vi "SQL_writeV2.vi"() -> ()   [LabVIEW 2019]
uses:
  <vilib>/OPCUA/NI OPC UA Client.lvlib
panel:
  out "date/time string":string
  in  "stop":bool
  in  "server endpoint URL":string
  # "OPC-UA Settings"
  # "SQL-Write Settings"
  # "Inputs:"
  # "Outputs"
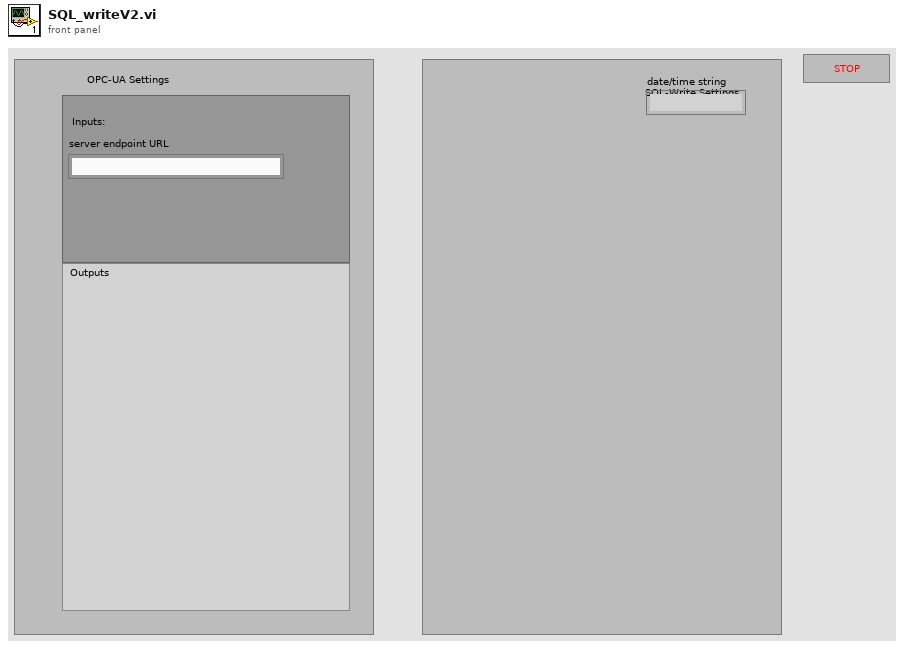
[diagram p1: front panel]
types:
  T1 = cluster{"message mode":enum16{"None", "Sign", "Sign and Encrypt"}, "security":enum16{"Basic256", "Basic128Rsa15"}}
  T2 = typedef "OPC UA Client Refnum.ctl" = refnum<k21>
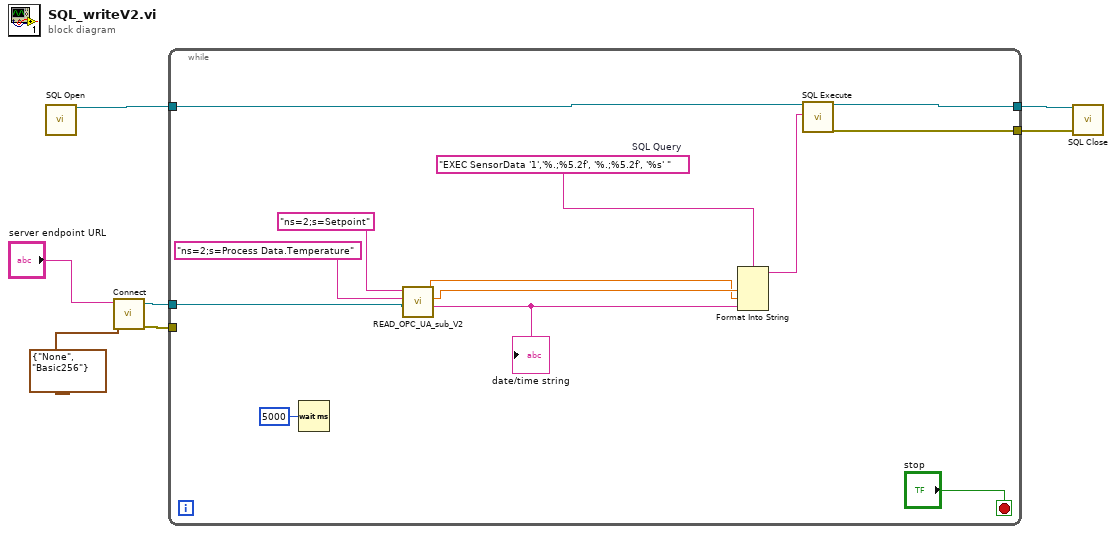
[diagram p0: block diagram]
diagram:
  n1 = call <vilib>:"SQL Open.vi"() -> ("ConnectionString In"=w2:string, "Connection Out"=w8:refnum<k7>)  [unwired: 17 in, 1 out]
  n2 = call <vilib>:"Connect.vi"("security policy"=T1 {"message mode"=enum."None", "security"=enum."Basic256"}, "server endpoint URL"="server endpoint URL") -> ("error out"=w3:errorcluster, "OPC UA client refnum out"=w4:T2)  [unwired: 7 in, 1 out]
  n3 = while {
    tunnel: w8 -> [w14]
    tunnel: [w13] -> w7
    tunnel: w4 -> [w17]
    tunnel: w3 -> [_]
    tunnel: [w12] -> w1
    stop <- "stop" stop-if-true
    w15 = "EXEC SensorData '1','%.;%5.2f', '%.;%5.2f', '%s' "  # SQL Query
    n4 = Wait (ms)(milliseconds to wait=u32 5000) -> ()  [unwired: 1 out]
    n5 = call "READ_OPC_UA_sub_V2.vi"("Node Id(setpoint)"="ns=2;s=Setpoint", "Node Id(temperature)"="ns=2;s=Process Data.Temperature", "OPC UA client refnum in"=w17) -> ("Temperature Value[C]"=w10:dbl, "Setpoint[C]"=w11:dbl, "date/time string"=w9:string)  [unwired: 5 in]
    "date/time string" <- w9
    n6 = Format Into String(format string=w15, w11, w10, w9) -> (resulting string=w16:string)  [unwired: 2 in, 1 out]
    n7 = call <vilib>:"SQL Execute.vi"("Connection In"=w14, "SQL Query"=w16) -> ("Connection Out"=w13:refnum<k7>, "Error out"=w12:errorcluster)  [unwired: 16 in]
  }
  n8 = call <vilib>:"SQL Close.vi"("Connection In"=w7, "Error in (no error)"=w1) -> ()  [unwired: 17 in, 1 out]
